vi "Variant_Set_TS_Propss_LV2015.vi"(6 "Insert If Missing":bool, 8 "error in (no error)":errorcluster, 9 "TS Paramter Ref Str":string="Step.Parameters", 10 "Sequence Context In":refnum<k7>, 11 "Parameters In":variant) -> (0 "error out":errorcluster, 2 "Sequence Context out":refnum<k7>)   [LabVIEW 2015]
uses:
  <vilib>/addons/TestStand/_TSUtility.llb/TestStand - Set Property Value (Number {Signed 8-bit Integer}).vi
  <vilib>/addons/TestStand/_TSUtility.llb/TestStand - Set Property Value (Number {Signed 16-bit Integer}).vi
  <vilib>/addons/TestStand/_TSUtility.llb/TestStand - Set Property Value (Number {Signed 32-bit Integer}).vi
  <vilib>/addons/TestStand/_TSUtility.llb/TestStand - Set Property Value (Number {Signed 64-bit Integer}).vi
  <vilib>/addons/TestStand/_TSUtility.llb/TestStand - Set Property Value (Number {Unsigned 8-bit Integer}).vi
  <vilib>/addons/TestStand/_TSUtility.llb/TestStand - Set Property Value (Number {Unsigned 16-bit Integer}).vi
  <vilib>/addons/TestStand/_TSUtility.llb/TestStand - Set Property Value (Number {Unsigned 32-bit Integer}).vi
  <vilib>/addons/TestStand/_TSUtility.llb/TestStand - Set Property Value (Number {Unsigned 64-bit Integer}).vi
  <vilib>/addons/TestStand/_TSUtility.llb/TestStand - Set Property Value (Number).vi
  <vilib>/addons/TestStand/_TSUtility.llb/TestStand - Set Property Value (Boolean).vi
  <vilib>/addons/TestStand/_TSUtility.llb/TestStand - Set Property Value (String).vi
  <vilib>/addons/TestStand/_TSUtility.llb/TestStand - Set Property Value (Reference).vi
panel:
  # "Connector Pane"
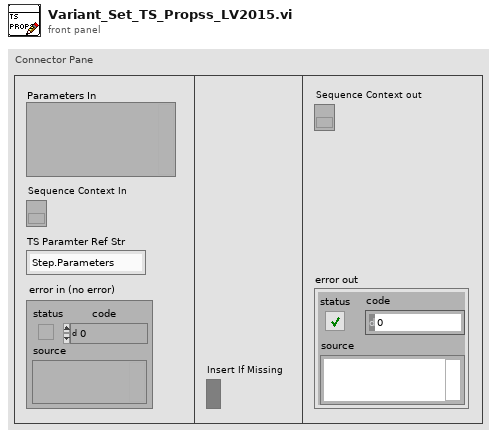
[diagram p1: front panel]
types:
  T1 = typedef "Type Descriptor Enumeration__ogtk.ctl" = enum8{"<Null>", "I8", "I16", "I32", "I64", "U8", "U16", "U32", "U64", "SGL", "DBL", "EXT", "CSG", "CDB", "CXT", "0x0F", "0x10", "0x11", "0x12", "0x13", "0x14", "Enum U8", "Enum U16", "Enum U32", "Enum U64", "SGL PQ", "DBL PQ", "EXT PQ", "CSG PQ", "CDB PQ", "CXT PQ", "0x1F", "0x20", "Boolean", "0x22", "0x23", "0x24", "0x25", "0x26", "0x27", "0x28", "0x29", "0x2A", "0x2B", "0x2C", "0x2D", "0x2E", "0x2F", "String", "0x31", "Path", "Pict", "0x34", "0x35", "0x36", "DAQ", "0x38", "0x39", "0x3A", "0x3B", "0x3C", "0x3D", "0x3E", "0x3F", "Array", "0x41", "0x42", "0x43", "0x44", "0x45", "0x46", "0x47", "0x48", "0x49", "0x4A", "0x4B", "0x4C", "0x4D", "0x4E", "0x4F", "Cluster", "0x51", "0x52", "Variant", "Waveform", "0x55", "0x56", "0x57", "0x58", "0x59", "0x5A", "0x5B", "0x5C", "0x5D", "0x5E", "0x5F", "0x60", "0x61", "0x62", "0x63", "0x64", "0x65", "0x66", "0x67", "0x68", "0x69", "0x6A", "0x6B", "0x6C", "0x6D", "0x6E", "0x6F", "Refnum"}
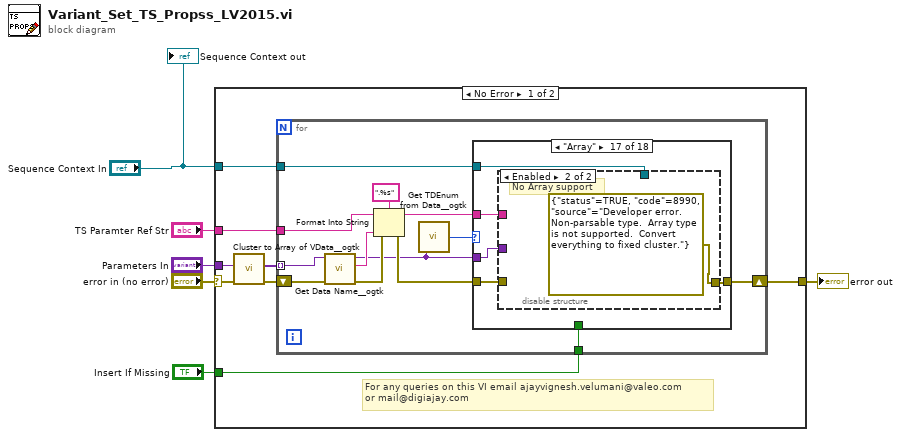
[diagram p0: block diagram]
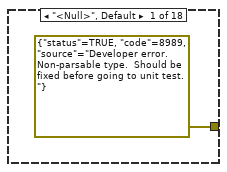
[diagram p2: hidden frame]
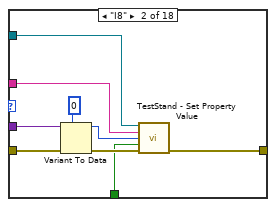
[diagram p3: hidden frame]
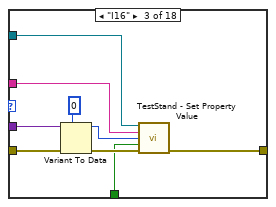
[diagram p4: hidden frame]
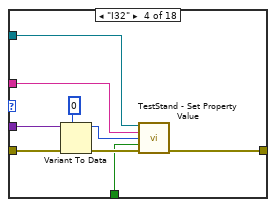
[diagram p5: hidden frame]
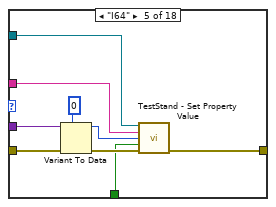
[diagram p6: hidden frame]
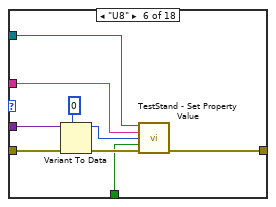
[diagram p7: hidden frame]
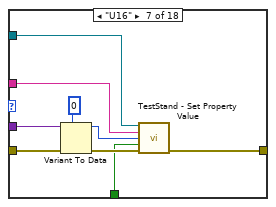
[diagram p8: hidden frame]
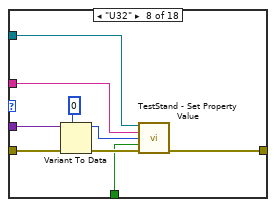
[diagram p9: hidden frame]
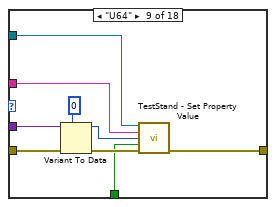
[diagram p10: hidden frame]
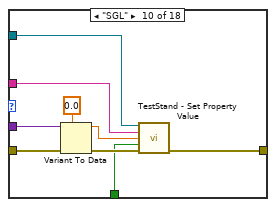
[diagram p11: hidden frame]
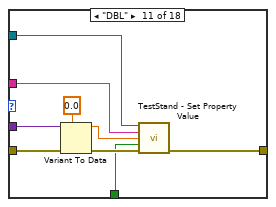
[diagram p12: hidden frame]
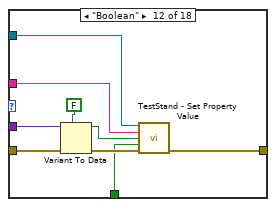
[diagram p13: hidden frame]
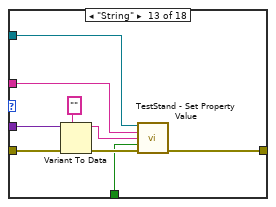
[diagram p14: hidden frame]
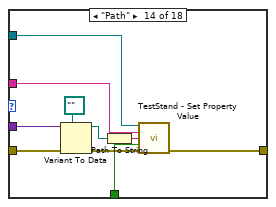
[diagram p15: hidden frame]
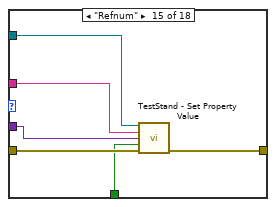
[diagram p16: hidden frame]
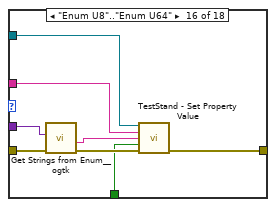
[diagram p17: hidden frame]
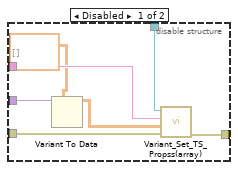
[diagram p18: hidden frame]
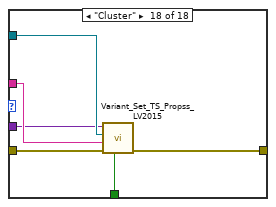
[diagram p19: hidden frame]
diagram:
  n1 = case shown="No Error" "error in (no error)" {
    selector: "error in (no error)" -> [w11 w180]
    tunnel: "Parameters In" -> [w14 _]
    tunnel: [w10 w180] -> w4
    tunnel: "TS Paramter Ref Str" -> [w9 _]
    tunnel: "Sequence Context In" -> [w8 _]
    tunnel: "Insert If Missing" -> [w7 _]
    frame No Error {
      # "For any queries on this VI email ajayvignesh.velumani@valeo.com\nor mail@digiajay.com"
      n2 = call <userlib>:"Cluster to Array of VData__ogtk.vi"("error in (no error)"=w11, "Cluster"=w14) -> ("error out"=w12:errorcluster, "Array of VData"=w13:variant[])  [unwired: 8 in]
      n3 = for {
        tunnel: w13 -> [w27] mode=indexing
        shift-right: [w25] -> w10
        shift-left: w12 -> [w26]
        tunnel: w9 -> [w20]
        tunnel: w8 -> [w17]
        tunnel: w7 -> [w15]
        n4 = call <userlib>:"Get Data Name__ogtk.vi"("error in (no error)"=w26, "Data"=w27) -> ("error out"=w23:errorcluster, "Data Name"=w19:string, "Data dup"=w16:variant)  [unwired: 7 in]
        n5 = Format Into String(format string=".%s", initial string=w20, error in=w23, w19) -> (resulting string=w18:string, error out=w22:errorcluster)
        n6 = call <userlib>:"Get TDEnum from Data__ogtk.vi"("Data"=w16) -> ("Type Descriptor Enumeration"=w24:T1)  [unwired: 4 in]
        n7 = case shown="\"Array\"" w24 {
          tunnel: [errorcluster {"status"=TRUE, "code"=8989, "source"="Developer error.  Non-parsable type.  Should be fixed before going to unit test."} ("error out") w37 w46 w55 w64 w73 w82 w91 w100 w109 w118 w127 w136 w146 w152 w160 w164 w178] -> w25
          tunnel: w22 -> [_ w36 w45 w54 w63 w72 w81 w90 w99 w108 w117 w126 w135 w145 w151 w157 w165 w179]
          tunnel: w18 -> [_ w35 w44 w53 w62 w71 w80 w89 w98 w107 w116 w125 w134 w144 w150 w159 w162 w177]
          tunnel: w16 -> [_ w33 w42 w51 w60 w69 w78 w87 w96 w105 w114 w123 w132 w142 w148 w156 w161 w175]
          tunnel: w17 -> [_ w30 w39 w48 w57 w66 w75 w84 w93 w102 w111 w120 w129 w140 w149 w158 w163 w176]
          tunnel: w15 -> [_ w29 w38 w47 w56 w65 w74 w83 w92 w101 w110 w119 w128 w137 w147 w153 _ w174]
          frame "<Null>", Default {
          }
          frame "I8" {
            n8 = Variant To Data(error in=w36, type=i8 0 ("New Value"), Variant=w33) -> (data=w31:i8, error out=w34:errorcluster)
            n9 = call-poly <vilib>:"TestStand - Set Property Value.vi"("Sequence Context In"=w30, "Lookup String"=w35, "New Value"=w31, "Insert If Missing"=w29, "error in (no error)"=w34) -> ("error out"=w37:errorcluster)  [unwired: 9 in, 1 out]
          }
          frame "I16" {
            n10 = Variant To Data(error in=w45, type=i16 0 ("New Value"), Variant=w42) -> (data=w40:i16, error out=w43:errorcluster)
            n11 = call-poly <vilib>:"TestStand - Set Property Value.vi"("Sequence Context In"=w39, "Lookup String"=w44, "New Value"=w40, "Insert If Missing"=w38, "error in (no error)"=w43) -> ("error out"=w46:errorcluster)  [unwired: 9 in, 1 out]
          }
          frame "I32" {
            n12 = Variant To Data(error in=w54, type=0 ("New Value"), Variant=w51) -> (data=w49:i32, error out=w52:errorcluster)
            n13 = call-poly <vilib>:"TestStand - Set Property Value.vi"("Sequence Context In"=w48, "Lookup String"=w53, "New Value"=w49, "Insert If Missing"=w47, "error in (no error)"=w52) -> ("error out"=w55:errorcluster)  [unwired: 9 in, 1 out]
          }
          frame "I64" {
            n14 = Variant To Data(error in=w63, type=i64 0 ("New Value"), Variant=w60) -> (data=w58:i64, error out=w61:errorcluster)
            n15 = call-poly <vilib>:"TestStand - Set Property Value.vi"("Sequence Context In"=w57, "Lookup String"=w62, "New Value"=w58, "Insert If Missing"=w56, "error in (no error)"=w61) -> ("error out"=w64:errorcluster)  [unwired: 9 in, 1 out]
          }
          frame "U8" {
            n16 = Variant To Data(error in=w72, type=u8 0 ("New Value"), Variant=w69) -> (data=w67:u8, error out=w70:errorcluster)
            n17 = call-poly <vilib>:"TestStand - Set Property Value.vi"("Sequence Context In"=w66, "Lookup String"=w71, "New Value"=w67, "Insert If Missing"=w65, "error in (no error)"=w70) -> ("error out"=w73:errorcluster)  [unwired: 9 in, 1 out]
          }
          frame "U16" {
            n18 = Variant To Data(error in=w81, type=u16 0 ("New Value"), Variant=w78) -> (data=w76:u16, error out=w79:errorcluster)
            n19 = call-poly <vilib>:"TestStand - Set Property Value.vi"("Sequence Context In"=w75, "Lookup String"=w80, "New Value"=w76, "Insert If Missing"=w74, "error in (no error)"=w79) -> ("error out"=w82:errorcluster)  [unwired: 9 in, 1 out]
          }
          frame "U32" {
            n20 = Variant To Data(error in=w90, type=u32 0 ("New Value"), Variant=w87) -> (data=w85:u32, error out=w88:errorcluster)
            n21 = call-poly <vilib>:"TestStand - Set Property Value.vi"("Sequence Context In"=w84, "Lookup String"=w89, "New Value"=w85, "Insert If Missing"=w83, "error in (no error)"=w88) -> ("error out"=w91:errorcluster)  [unwired: 9 in, 1 out]
          }
          frame "U64" {
            n22 = Variant To Data(error in=w99, type=u64 0 ("New Value"), Variant=w96) -> (data=w94:u64, error out=w97:errorcluster)
            n23 = call-poly <vilib>:"TestStand - Set Property Value.vi"("Sequence Context In"=w93, "Lookup String"=w98, "New Value"=w94, "Insert If Missing"=w92, "error in (no error)"=w97) -> ("error out"=w100:errorcluster)  [unwired: 9 in, 1 out]
          }
          frame "SGL" {
            n24 = Variant To Data(error in=w108, type=0.0 ("New Value"), Variant=w105) -> (data=w103:dbl, error out=w106:errorcluster)
            n25 = call-poly <vilib>:"TestStand - Set Property Value.vi"("Sequence Context In"=w102, "Lookup String"=w107, "New Value"=w103, "Insert If Missing"=w101, "error in (no error)"=w106) -> ("error out"=w109:errorcluster)  [unwired: 9 in, 1 out]
          }
          frame "DBL" {
            n26 = Variant To Data(error in=w117, type=0.0 ("New Value"), Variant=w114) -> (data=w112:dbl, error out=w115:errorcluster)
            n27 = call-poly <vilib>:"TestStand - Set Property Value.vi"("Sequence Context In"=w111, "Lookup String"=w116, "New Value"=w112, "Insert If Missing"=w110, "error in (no error)"=w115) -> ("error out"=w118:errorcluster)  [unwired: 9 in, 1 out]
          }
          frame "Boolean" {
            n28 = Variant To Data(error in=w126, type=FALSE, Variant=w123) -> (data=w121:bool, error out=w124:errorcluster)
            n29 = call-poly <vilib>:"TestStand - Set Property Value.vi"("Sequence Context In"=w120, "Lookup String"=w125, "New Value"=w121, "Insert If Missing"=w119, "error in (no error)"=w124) -> ("error out"=w127:errorcluster)  [unwired: 9 in, 1 out]
          }
          frame "String" {
            n30 = Variant To Data(error in=w135, type="", Variant=w132) -> (data=w130:string, error out=w133:errorcluster)
            n31 = call-poly <vilib>:"TestStand - Set Property Value.vi"("Sequence Context In"=w129, "Lookup String"=w134, "New Value"=w130, "Insert If Missing"=w128, "error in (no error)"=w133) -> ("error out"=w136:errorcluster)  [unwired: 9 in, 1 out]
          }
          frame "Path" {
            n32 = Variant To Data(error in=w145, type=path "", Variant=w142) -> (data=w139:path, error out=w143:errorcluster)
            n33 = Path To String(path=w139) -> (string=w138:string)
            n34 = call-poly <vilib>:"TestStand - Set Property Value.vi"("Sequence Context In"=w140, "Lookup String"=w144, "New Value"=w138, "Insert If Missing"=w137, "error in (no error)"=w143) -> ("error out"=w146:errorcluster)  [unwired: 9 in, 1 out]
          }
          frame "Refnum" {
            n35 = call-poly <vilib>:"TestStand - Set Property Value.vi"("Sequence Context In"=w149, "Lookup String"=w150, "New Value"=w148, "Insert If Missing"=w147, "error in (no error)"=w151) -> ("error out"=w152:errorcluster)  [unwired: 9 in, 1 out]
          }
          frame "Enum U8".."Enum U64" {
            n36 = call <userlib>:"Get Strings from Enum__ogtk.vi"("error in (no error)"=w157, "Enum"=w156) -> ("error out"=w155:errorcluster, "String Value"=w154:string)  [unwired: 6 in, 2 out]
            n37 = call-poly <vilib>:"TestStand - Set Property Value.vi"("Sequence Context In"=w158, "Lookup String"=w159, "New Value"=w154, "Insert If Missing"=w153, "error in (no error)"=w155) -> ("error out"=w160:errorcluster)  [unwired: 9 in, 1 out]
          }
          frame "Array" {
            n38 = disable-structure shown="Enabled" {
              disable-tunnel: w165 -> [w172 _]
              disable-tunnel: [w171 errorcluster {"status"=TRUE, "code"=8990, "source"="Developer error.  Non-parsable type.  Array type  is not supported.  Convert everything to fixed cluster."} ("error out")] -> w164
              disable-tunnel: w163 -> [w170 _]
              disable-tunnel: w162 -> [w169 _]
              disable-tunnel: w161 -> [w168 _]
              frame Disabled {
                n39 = Variant To Data(type=dbl[][] [], Variant=w168) -> (data=w167:dbl[][])  [unwired: 1 in, 1 out]
                n40 = call "Variant_Set_TS_Propss(array).vi"("error in (no error)"=w172, "newValue"=w167, "lookupString"=w169, "Automation Refnum in"=w170) -> ("error out"=w171:errorcluster)  [unwired: 7 in]
              }
              frame Enabled {
                # "No Array support"
              }
            }
          }
          frame "Cluster" {
            n41 = call "Variant_Set_TS_Propss_LV2015.vi"("Insert If Missing"=w174, "error in (no error)"=w179, "TS Paramter Ref Str"=w177, "Sequence Context In"=w176, "Parameters In"=w175) -> ("error out"=w178:errorcluster)  [unwired: 5 in, 1 out]
          }
        }
      }
    }
    frame Error {
    }
  }
  "error out" <- w4
  "Sequence Context out" <- "Sequence Context In"
